vi "Draw.vi"(1 "Grids":i32[][](array[numeric]), 2 "Picture in":refnum<vi>) -> (0 "reference out":refnum<vi>)   [LabVIEW 2018]
doc: "Draw a picture on GridsPic."
panel:
  in  "GridPicture":T1(array[cluster])=[{"type"=0, "depth"=24, "image"=array[19200 elements], "mask"=[], "colors"=[], "Rectangle"={"left"=0, "top"=0, "right"=80, "bottom"=80}}, {"type"=0, "depth"=24, "image"=array[19200 elements], "mask"=[], "colors"=[], "Rectangle"={"left"=0, "top"=0, "right"=80, "bottom"=80}}, {"type"=0, "depth"=24, "image"=array[19200 elements], "mask"=[], "colors"=[], "Rectangle"={"left"=0, "top"=0, "right"=80, "bottom"=80}}, {"type"=0, "depth"=24, "image"=array[19200 elements], "mask"=[], "colors"=[], "Rectangle"={"left"=0, "top"=0, "right"=80, "bottom"=80}}, {"type"=0, "depth"=24, "image"=array[19200 elements], "mask"=[], "colors"=[], "Rectangle"={"left"=0, "top"=0, "right"=80, "bottom"=80}}, {"type"=0, "depth"=24, "image"=array[19200 elements], "mask"=[], "colors"=[], "Rectangle"={"left"=0, "top"=0, "right"=80, "bottom"=80}}, {"type"=0, "depth"=24, "image"=array[19200 elements], "mask"=[], "colors"=[], "Rectangle"={"left"=0, "top"=0, "right"=80, "bottom"=80}}, {"type"=0, "depth"=24, "image"=array[19200 elements], "mask"=[], "colors"=[], "Rectangle"={"left"=0, "top"=0, "right"=80, "bottom"=80}}, {"type"=0, "depth"=24, "image"=array[19200 elements], "mask"=[], "colors"=[], "Rectangle"={"left"=0, "top"=0, "right"=80, "bottom"=80}}, {"type"=0, "depth"=24, "image"=array[19200 elements], "mask"=[], "colors"=[], "Rectangle"={"left"=0, "top"=0, "right"=80, "bottom"=80}}, {"type"=0, "depth"=24, "image"=array[19200 elements], "mask"=[], "colors"=[], "Rectangle"={"left"=0, "top"=0, "right"=80, "bottom"=80}}, {"type"=0, "depth"=24, "image"=array[19200 elements], "mask"=[], "colors"=[], "Rectangle"={"left"=0, "top"=0, "right"=80, "bottom"=80}}, {"type"=0, "depth"=24, "image"=array[19200 elements], "mask"=[], "colors"=[], "Rectangle"={"left"=0, "top"=0, "right"=80, "bottom"=80}}, {"type"=0, "depth"=24, "image"=array[19200 elements], "mask"=[], "colors"=[], "Rectangle"={"left"=0, "top"=0, "right"=80, "bottom"=80}}, {"type"=0, "depth"=24, "image"=array[19200 elements], "mask"=[], "colors"=[], "Rectangle"={"left"=0, "top"=0, "right"=80, "bottom"=80}}, {"type"=0, "depth"=24, "image"=array[19200 elements], "mask"=[], "colors"=[], "Rectangle"={"left"=0, "top"=0, "right"=80, "bottom"=80}}, {"type"=0, "depth"=24, "image"=array[19200 elements], "mask"=[], "colors"=[], "Rectangle"={"left"=0, "top"=0, "right"=80, "bottom"=80}}, {"type"=0, "depth"=24, "image"=array[19200 elements], "mask"=[], "colors"=[], "Rectangle"={"left"=0, "top"=0, "right"=80, "bottom"=80}}]
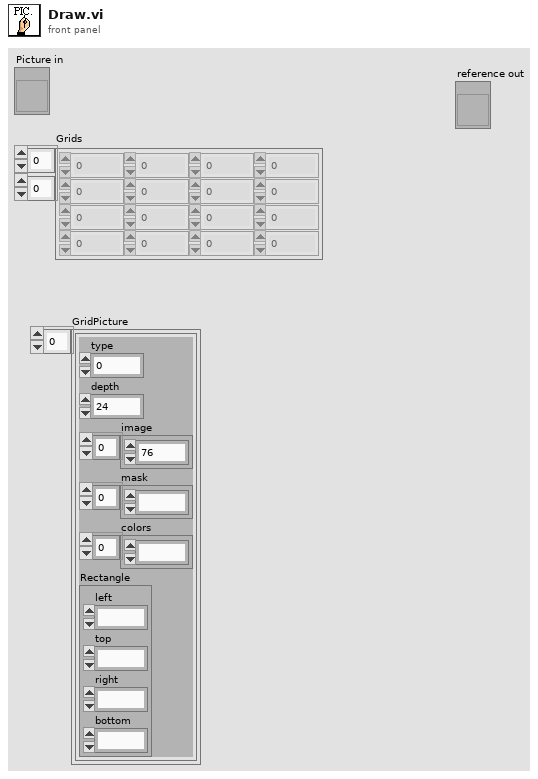
[diagram p1: front panel]
types:
  T1 = cluster{"type":i32, "depth":i32, "image":u8[], "mask":u8[], "colors":u32[], "Rectangle":cluster{"left":i16, "top":i16, "right":i16, "bottom":i16}}[]
  T2 = cluster{"type":i32, "depth":i32, "image":u8[], "mask":u8[], "colors":u32[], "Rectangle":cluster{"left":i16, "top":i16, "right":i16, "bottom":i16}}
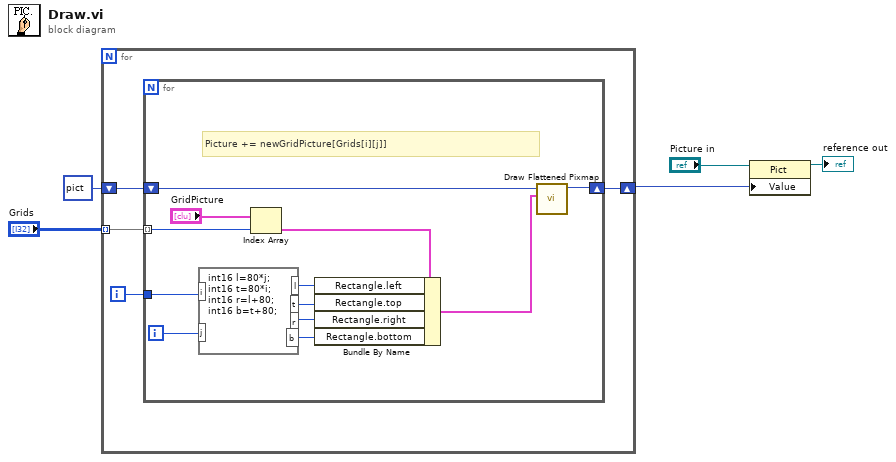
[diagram p0: block diagram]
diagram:
  n1 = for {
    tunnel: "Grids" -> [w9] mode=indexing
    shift-right: [w7] -> w2
    shift-left: picture data[5B] ("new picture") -> [w8]
    i -> [w6]
    n2 = for {
      tunnel: w9 -> [w20] mode=indexing
      shift-right: [w18] -> w7
      shift-left: w8 -> [w19]
      tunnel: w6 -> [w11]
      i -> [w10]
      # "Picture += newGridPicture[Grids[i][j]]"
      n3 = formula code="int16 l=80*j;\nint16 t=80*i;\nint16 r=l+80;\nint16 b=t+80;"("i"=w11, "j"=w10) -> ("l"=w17:i16, "t"=w16:i16, "r"=w15:i16, "b"=w14:i16)
      n4 = Index Array(array="GridPicture", index=w20) -> (element=w13:T2)
      n5 = Bundle By Name(cluster=w13, "Rectangle.left"=w17, "Rectangle.top"=w16, "Rectangle.right"=w15, "Rectangle.bottom"=w14) -> (w12:T2)
      n6 = call <vilib>:"Draw Flattened Pixmap.vi"("image data"=w12, "picture"=w19) -> ("new picture"=w18:picture)  [unwired: 7 in]
    }
  }
  n7 = property class="Pict"(reference="Picture in", "Value"=w2) -> (reference out=→"reference out":refnum<vi>)  [unwired: 1 in, 1 out]
